vi "Length Delimited Encoder.vi"(9 "Array In":u8[](array[numeric]), 10 "Key":u32, 11 "Array In 2":u8[](array[numeric])) -> (1 "Array":u8[](array[numeric]))   [LabVIEW 2018]
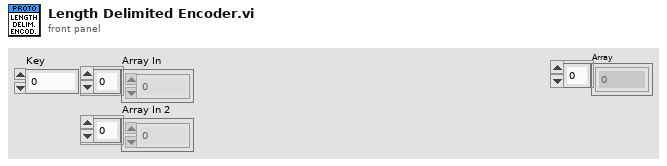
[diagram p1: front panel]
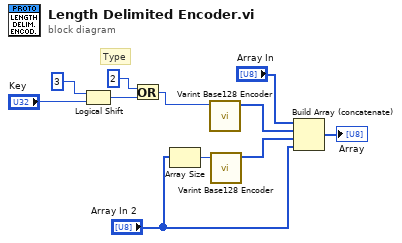
[diagram p0: block diagram]
diagram:
  # "Type"
  n1 = Logical Shift(y=i16 3, x="Key") -> (x << y=w9:u32)
  n2 = Or(x=u32 2, y=w9) -> (x .or. y?=w7:u32)
  n3 = Array Size(array="Array In 2") -> (size(s)=w2:i32)
  n4 = call "Varint Base128 Encoder.vi"("Numeric"=w7) -> ("Array"=w6:u8[])  [unwired: 10 in]
  n5 = call "Varint Base128 Encoder.vi"("Numeric"=w2) -> ("Array"=w5:u8[])  [unwired: 10 in]
  n6 = Build Array (concatenate)("Array In", w6, w5, "Array In 2") -> (→"Array":u8[])
